vi "PFI-28000-Utils_Parse Channel Info.vi"(0 "String":string, 11 "error in (no error)":errorcluster) -> (4 "Channel Count":i32, 6 "Channels per Card":i32, 15 "error out":errorcluster)   [LabVIEW 2017, in "PFI-28000-Utils.lvlib"]
uses:
  PFI-28000-Utils.lvlib
  <vilib>/regexp/Match Regular Expression.xnode
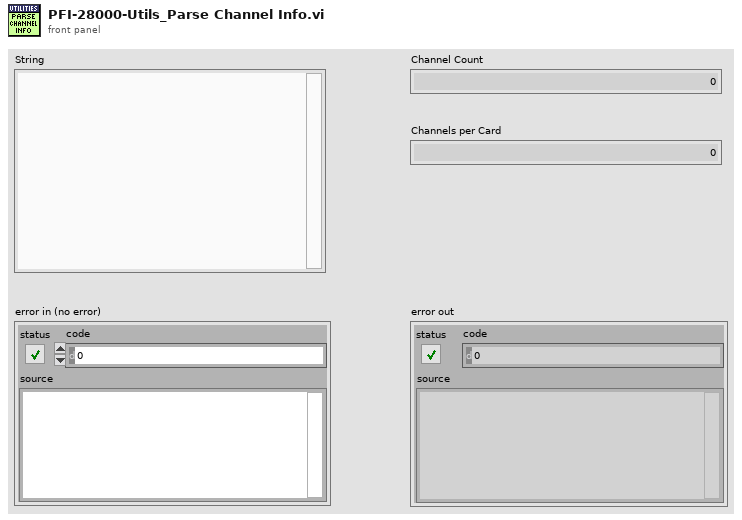
[diagram p1: front panel]
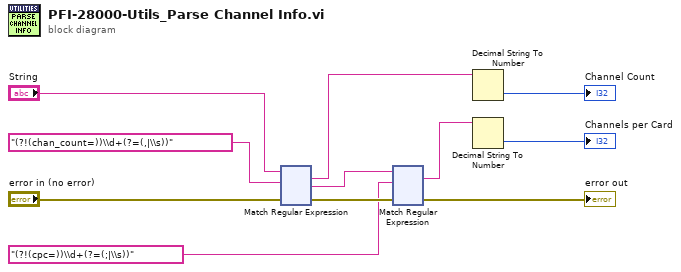
[diagram p0: block diagram]
diagram:
  n1 = xnode "Match Regular Expression"("input string"="String", "regular expression"="(?!(chan_count=))\\d+(?=(,|\\s))" ("empty string"), "error in"="error in (no error)") -> ("whole match"=w2:string, "after match"=w8:string, "error out"=w6:errorcluster)  [unwired: 3 in, 2 out]
  n2 = xnode "Match Regular Expression"("input string"=w8, "regular expression"="(?!(cpc=))\\d+(?=(;|\\s))" ("empty string"), "error in"=w6) -> ("whole match"=w7:string, "error out"=→"error out":errorcluster)  [unwired: 3 in, 3 out]
  n3 = Decimal String To Number(string=w2) -> (number=→"Channel Count":i32)  [unwired: 2 in, 1 out]
  n4 = Decimal String To Number(string=w7) -> (number=→"Channels per Card":i32)  [unwired: 2 in, 1 out]
